vi "test_Tx Exec Unit (Generic).vi"() -> ()   [LabVIEW 2020]
uses:
  Shared/hardware_channels_tx.ctl
  Shared/channel_settings_tx.ctl
  Shared/Frame Payload Parameters.ctl
  Shared/Encoding (Arinc664).ctl
  Shared/RawFrame_entry.ctl
  <instrlib>/AIM GmbH/_AIM 664/_controls/queue_header_generic.ctl
  Engine/Interfaces/Shared Resources/Shared Resources.lvclass
  <vilib>/NI VeriStand/Custom Device API/Custom Device Item Ref.ctl
  Engine/Implementation/Tx Execution Unit/Tx Generic Execution Unit.lvclass
  <vilib>/NI VeriStand/Custom Device API/Custom Device API.lvlib
  <instrlib>/AIM GmbH/_AIM 664/AIM664LV.lvlib
panel:
  in  "Update data every N calls":i32=1
  out "Read Time (us)":u32
  out "Tx Gen Execution Speed":u32(graph)
  out "Write Time (us)":u32
  in  "from file":bool
  in  "Values in":dbl[](array[numeric])=[1.0, 1.0, 1.0]
  in  "enable tx":bool=TRUE
  out "Frame parse error":errorcluster caption="error out"
  in  "file path (use dialog)":path=path "/home/admin/Tx_Gen_Config.bin"
  out "Values out":dbl[](array[numeric])
  in  "TX Parameters":T1={"channel #"=0, "channel handle"=0, "InstrumentHandle_board"=0, "InstrumentHandle_port"=0, "channel settings"={"Tx Board"=0, "Tx Port"=0, "Payload Parameter Array"=[{"PayloadID"="Payload1", "FrameIndeces"=[0], "Parameters"=[{"start index"=0, "size"=64, "encoding"=0, "signed"=TRUE, "scale multiplier"=1.0, "scale offset"=0.0}, {"start index"=64, "size"=64, "encoding"=0, "signed"=TRUE, "scale multiplier"=1.0, "scale offset"=0.0}]}], "QueueSizeIn"=0, "Count"=0, "StartMode"=1}, "PayloadMap"={"Payload1"=[3, 0, 0, 0, 0, 60, 2, 0, 0, 1, 33, 32, 8, 0, 69, 0, 0, 60, 0, 0, 64, 0, 1, 17, 109, 147, 10, 1, 33, 1, 224, 224, 0, 60, 0, 23, 0, 24, 0, 40, 0, 0, 0, 0, 0, 0, 0, 0, 0, 0, 0, 0, 0, 0, 0, 0, 0, 0, 0, 0, 0, 0, 0, 0, 0, 0, 0, 0, 0, 0, 0, 0, 0, 0, 0, 0, 0, 0, 0]}, "RawFrameMap"={}} {"channel settings"."Payload Parameter Array"."Parameters"."encoding" items=["BNR", "BCD", "Discrete"]}
  out "error out":errorcluster
  in  "stop":bool
  in  "loop rate mS":u32=10
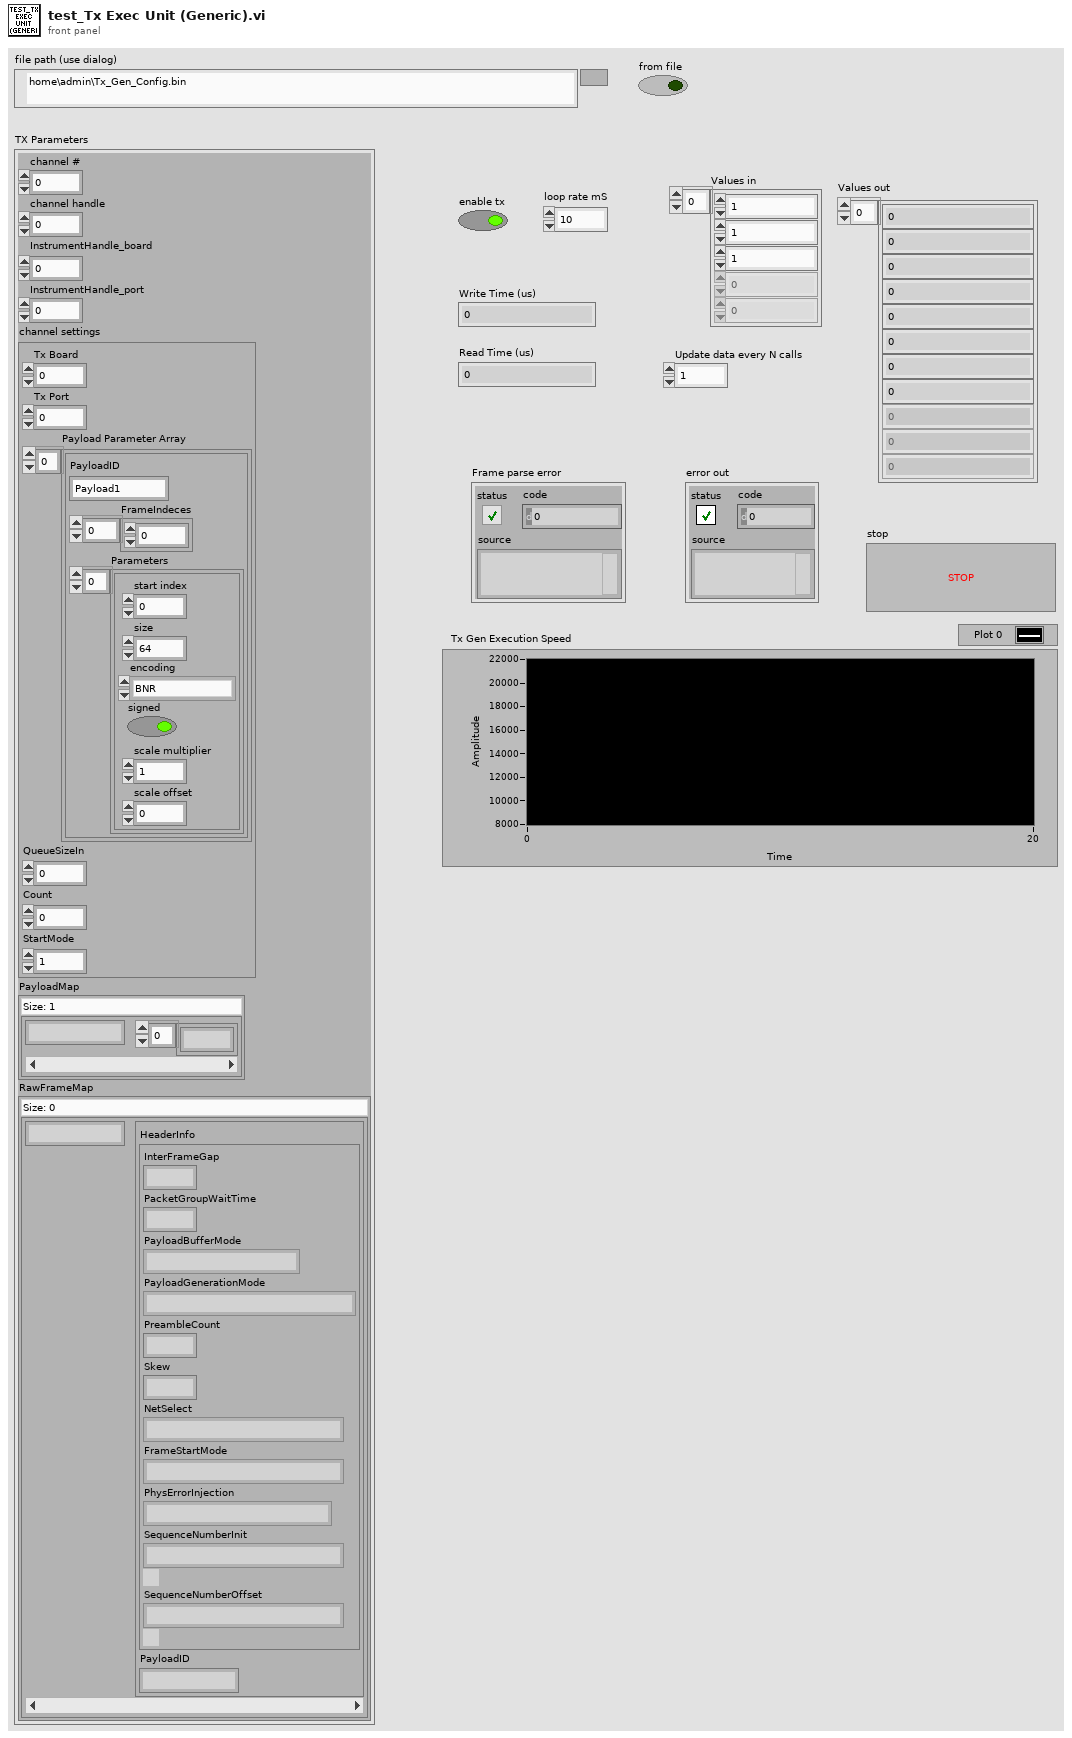
[diagram p1: front panel]
types:
  T1 = typedef "hardware_channels_tx.ctl" = cluster{"channel #":u16, "channel handle":u64, "InstrumentHandle_board":u32, "InstrumentHandle_port":u32, "channel settings":T2, "PayloadMap":map{string, u8[]}, "RawFrameMap":map{string, T5}}
  T2 = typedef "channel_settings_tx.ctl" = cluster{"Tx Board":u32, "Tx Port":u32, "Payload Parameter Array":T3[], "QueueSizeIn":u32, "Count":u32, "StartMode":u32}
  T3 = typedef "Frame Payload Parameters.ctl" = cluster{"PayloadID":string, "FrameIndeces":u32[], "Parameters":cluster{"start index":i32, "size":i32, "encoding":T4, "signed":bool, "scale multiplier":dbl, "scale offset":dbl}[]}
  T4 = typedef "Encoding (Arinc664).ctl" = u16
  T5 = typedef "RawFrame_entry.ctl" = cluster{"HeaderInfo":T6, "PayloadID":string}
  T6 = typedef "AIM664LV.lvlib/queue_header_generic.ctl" = cluster{"InterFrameGap":u32, "PacketGroupWaitTime":u32, "PayloadBufferMode":u8, "PayloadGenerationMode":u8, "PreambleCount":u8, "Skew":u32, "NetSelect":u8, "FrameStartMode":u8, "PhysErrorInjection":u32, "SequenceNumberInit":u16, "SequenceNumberOffset":u16}
  T7 = typedef "Custom Device API.lvlib/Custom Device Item Ref.ctl" = u64
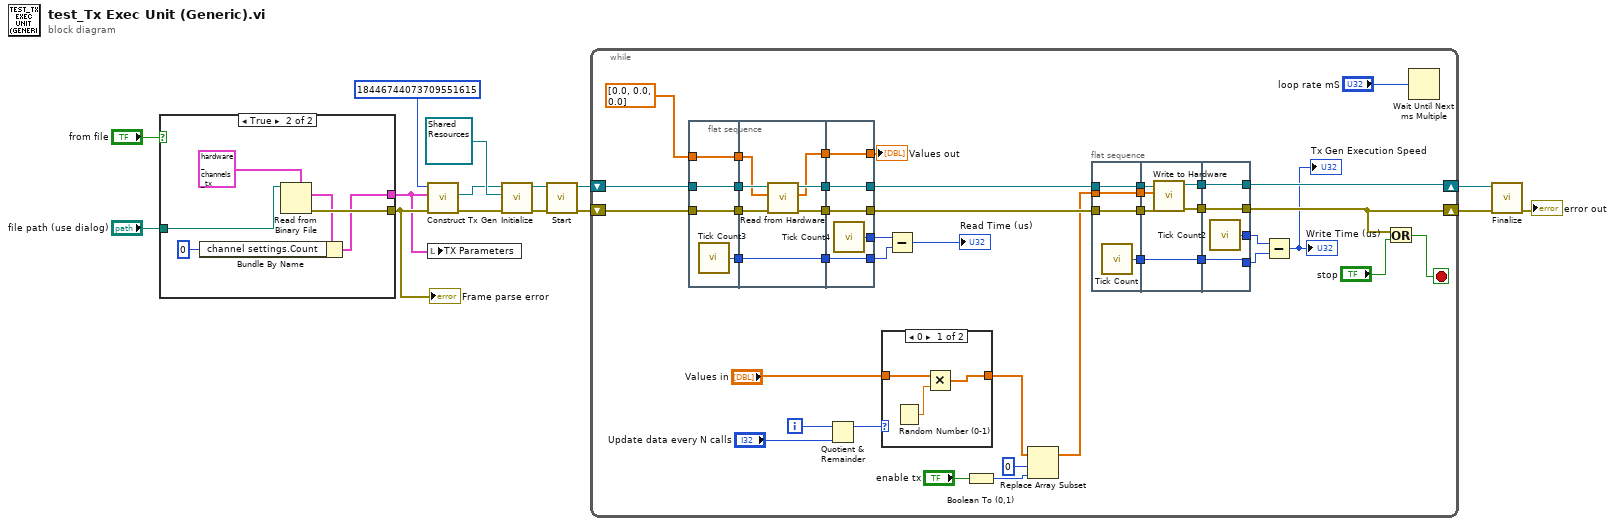
[diagram p0: block diagram]
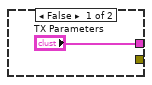
[diagram p2: hidden frame]
diagram:
  n1 = case shown="True" "from file" {
    tunnel: "file path (use dialog)" -> [_ w20]
    tunnel: [_ w22] -> w2
    tunnel: ["TX Parameters" w18] -> w1
    frame False {
    }
    frame True {
      n2 = Read from Binary File(5:T1 {"channel #"=0, "channel handle"=0, "InstrumentHandle_board"=0, "InstrumentHandle_port"=0, "channel settings"={"Tx Board"=0, "Tx Port"=0, "Payload Parameter Array"=[], "QueueSizeIn"=0, "Count"=0, "StartMode"=0}, "PayloadMap"={}, "RawFrameMap"={}} ("Tx cluster out"), 11:w20) -> (0:w22:errorcluster, 2:w17:T1)  [unwired: 4 in, 2 out]
      n3 = Bundle By Name(cluster=w17, "channel settings.Count"=u32 0) -> (w18:T1)
    }
  }
  "Frame parse error" <- w2
  n4 = call "Construct Tx Gen.vi"("error in (no error)"=w2, "TX Parameters"=w1, "custom device ref in"=T7 18446744073709551615) -> ("error out"=w6:errorcluster, "Tx Execution Unit out"=w7:refnum<class "Tx Generic Execution Unit.lvclass">)  [unwired: 5 in, 1 out]
  n5 = local write "TX Parameters"(w1) -> ()
  n6 = call-dynamic "Initialize.vi"("error in"=w6, "shared resources"=refnum<class "Shared Resources.lvclass"> refnum, "Tx Execution Unit Implementation in"=w7) -> ("error out"=w10:errorcluster, "Tx Execution Unit Implementation out"=w15:refnum<class "Tx Generic Execution Unit.lvclass">)  [unwired: 7 in]
  n7 = call-dynamic "Start.vi"("error in"=w10, "Tx Execution Unit Implementation in"=w15) -> ("error out"=w13:errorcluster, "Tx Execution Unit Implementation out"=w14:refnum<class "Tx Generic Execution Unit.lvclass">)  [unwired: 8 in]
  n8 = while {
    shift-right: [w59] -> w12
    shift-left: w14 -> [w63]
    shift-right: [w57] -> w11
    shift-left: w13 -> [w62]
    i -> [w27]
    stop <- w55 stop-if-true
    n9 = flat-sequence {
      tunnel: dbl[] [0.0, 0.0, 0.0] ("Values in") -> [w69]
      tunnel: w62 -> [w70]
      tunnel: w63 -> [w71]
      tunnel: [w71] -> w39
      tunnel: [w70] -> w38
      tunnel: [w69] -> w37
      tunnel: [w68] -> w30
      tunnel: w39 -> [w78]
      tunnel: w38 -> [w77]
      tunnel: w37 -> [w73]
      tunnel: [w76] -> w36
      tunnel: [w75] -> w35
      tunnel: [w74] -> w34
      tunnel: [w72] -> w31
      tunnel: w30 -> [w72]
      tunnel: [w81] -> w54
      tunnel: [w82] -> w60
      tunnel: [w83] -> w61
      tunnel: w36 -> [w83]
      tunnel: w35 -> [w82]
      tunnel: w34 -> [w81]
      tunnel: [w80] -> w33
      tunnel: [w79] -> w32
      tunnel: w31 -> [w79]
      frame #0 {
        n10 = call "Tick Count3"() -> ("Tick Count(uSec)"=w68:u32)
      }
      frame #1 {
        n11 = call-dynamic "Read from Hardware.vi"("error in"=w77, "Values in"=w73, "Tx Execution Unit Implementation in"=w78) -> ("error out"=w75:errorcluster, "Values out"=w74:dbl[], "Tx Execution Unit Implementation out"=w76:refnum<class "Tx Generic Execution Unit.lvclass">)  [unwired: 6 in]
      }
      frame #2 {
        n12 = call "Tick Count4"() -> ("Tick Count(uSec)"=w80:u32)
      }
    }
    n13 = Quotient & Remainder(x=w27, y="Update data every N calls") -> (x-y*floor(x/y)=w28:i32)  [unwired: 1 out]
    n14 = case shown="0" w28 {
      tunnel: "Values in" -> [w66 w67]
      tunnel: [w65 w67] -> w24
      frame 0 {
        n15 = Random Number (0-1)() -> (number: 0 to 1=w64:dbl)
        n16 = Multiply(x=w66, y=w64) -> (x*y=w65:dbl[])
      }
      frame 1, Default {
      }
    }
    n17 = Subtract(x=w33, y=w32) -> (x-y=→"Read Time (us)":u32)
    n18 = Boolean To (0,1)(Boolean="enable tx") -> (0, 1=w53:i16)
    n19 = Replace Array Subset(array=w24, new element=w53, index=0) -> (w23:dbl[])
    n20 = flat-sequence {
      tunnel: w23 -> [w85]
      tunnel: w60 -> [w86]
      tunnel: w61 -> [w87]
      tunnel: [w87] -> w47
      tunnel: [w86] -> w46
      tunnel: [w85] -> w45
      tunnel: [w84] -> w43
      tunnel: [w91] -> w49
      tunnel: [w90] -> w48
      tunnel: w47 -> [w93]
      tunnel: w46 -> [w92]
      tunnel: w45 -> [w89]
      tunnel: [w88] -> w44
      tunnel: w43 -> [w88]
      tunnel: [w96] -> w57
      tunnel: [w97] -> w59
      tunnel: w49 -> [w97]
      tunnel: w48 -> [w96]
      tunnel: [w95] -> w41
      tunnel: w44 -> [w95]
      tunnel: [w94] -> w42
      frame #0 {
        n21 = call "Tick Count"() -> ("Tick Count(uSec)"=w84:u32)
      }
      frame #1 {
        n22 = call-dynamic "Write to Hardware.vi"("error in"=w92, "Values in"=w89, "Tx Execution Unit Implementation in"=w93) -> ("error out"=w90:errorcluster, "Tx Execution Unit Implementation out"=w91:refnum<class "Tx Generic Execution Unit.lvclass">)  [unwired: 5 in, 2 out]
      }
      frame #2 {
        n23 = call "Tick Count2"() -> ("Tick Count(uSec)"=w94:u32)
      }
    }
    n24 = Subtract(x=w42, y=w41) -> (x-y=→"Write Time (us)" →"Tx Gen Execution Speed":u32)
    n25 = Or(x=w57, y="stop") -> (x .or. y?=w55:bool)
    n26 = Wait Until Next ms Multiple(millisecond multiple="loop rate mS") -> ()  [unwired: 1 out]
    "Values out" <- w54
  }
  n27 = call-dynamic "Finalize.vi"("error in"=w11, "Tx Execution Unit in"=w12) -> ("error out"=→"error out":errorcluster)  [unwired: 8 in, 1 out]
